vi "testReceiverStream.vi"() -> ()   [LabVIEW 2018]
uses:
  NetworkStreamData.ctl
  NetworkStream.lvlib
panel:
  out "data out":T1
  out "timed out?":bool
  in  "timeout ms (-1)":i32
  out "error out":errorcluster
  in  "stop":bool
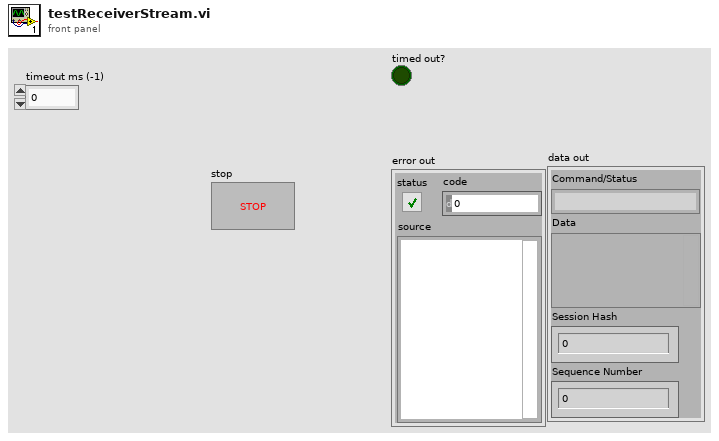
[diagram p1: front panel]
types:
  T1 = typedef "NetworkStream.lvlib/NetworkStreamData.ctl" = cluster{"Command/Status":string, "Data":variant, "Session Hash":u64, "Sequence Number":u64}
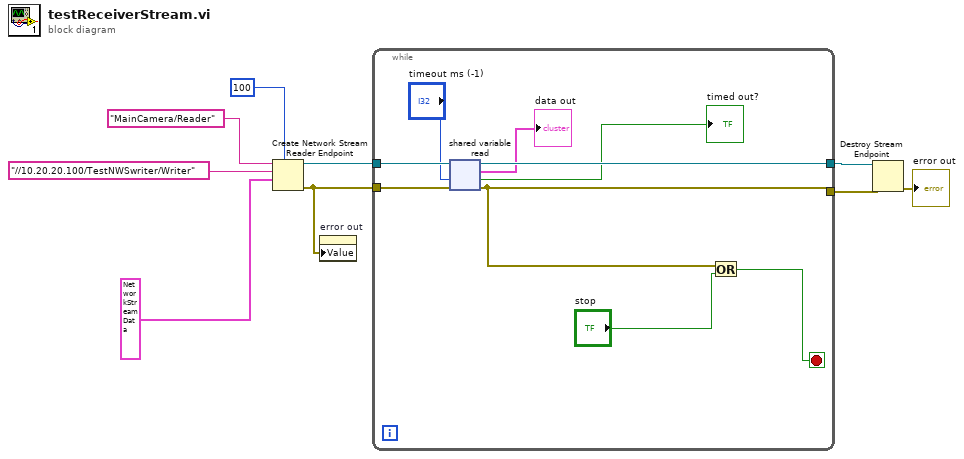
[diagram p0: block diagram]
diagram:
  (unwired) T1 {"Command/Status"="", "Data"=variant, "Session Hash"=0, "Sequence Number"=0} ("NetworkStreamCluster")
  n1 = Create Network Stream Reader Endpoint(7:100 ("reader buffer size"), 9:T1 {"Command/Status"="", "Data"=variant, "Session Hash"=0, "Sequence Number"=0} ("NetworkStreamCluster"), 10:"//10.20.20.100/TestNWSwriter/Writer" ("writer url"), 11:"MainCamera/Reader" ("reader name")) -> (0:w3:errorcluster, 3:w9:refnum<k21>)  [unwired: 3 in]
  n2 = property on="error out" class="Clust (strict)"("Value"=w3) -> ()  [unwired: 2 in, 2 out]
  n3 = while {
    tunnel: w9 -> [w18]
    tunnel: w3 -> [w17]
    tunnel: [w13] -> w7
    tunnel: [w15] -> w6
    stop <- w14 stop-if-true
    n4 = shared-variable-read(w18, w17, "timeout ms (-1)") -> (w15:refnum<k21>, w13:errorcluster, →"timed out?":bool, →"data out":T1)
    n5 = Or(x=w13, y="stop") -> (x .or. y?=w14:bool)
  }
  n6 = Destroy Stream Endpoint(8:w7, 11:w6) -> (0:→"error out":errorcluster)
